vi "ReadTerminal.vi"(1 "reference":refnum<vi>) -> (0 "Terminal":T4)   [LabVIEW 2013]
uses:
  <vilib>/Utility/miscctls.llb/LVBoundsTypeDef.ctl
  <vilib>/Utility/miscctls.llb/LVRectTypeDef.ctl
  <vilib>/Utility/miscctls.llb/LVPositionTypeDef.ctl
panel:
  out "error out":errorcluster
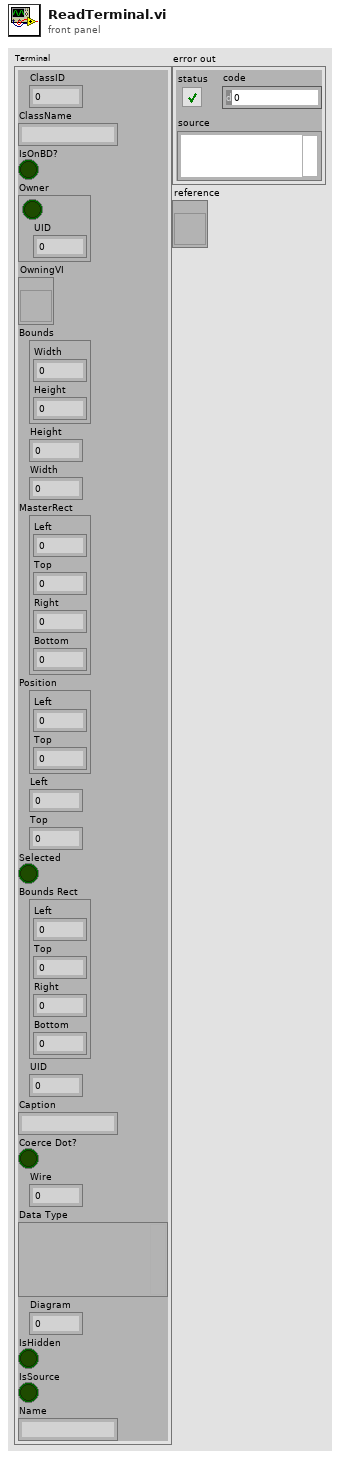
[diagram p1: front panel]
types:
  T1 = typedef "LVBoundsTypeDef.ctl" = cluster{"Width":u32, "Height":u32}
  T2 = typedef "LVRectTypeDef.ctl" = cluster{"Left":i16, "Top":i16, "Right":i16, "Bottom":i16}
  T3 = typedef "LVPositionTypeDef.ctl" = cluster{"Left":i32, "Top":i32}
  T4 = cluster{"ClassID":u32, "ClassName":string, "IsOnBD?":bool, "Owner":cluster{bool, "UID":i32}, "OwningVI":refnum<vi>, "Bounds":T1, "Height":u32, "Width":u32, "MasterRect":T2, "Position":T3, "Left":i32, "Top":i32, "Selected":bool, "Bounds Rect":T2, "UID":i32, "Caption":string, "Coerce Dot?":bool, "Wire":i32, "Data Type":variant, "Diagram":i32, "IsHidden":bool, "IsSource":bool, "Name":string}
  T5 = cluster{"ClassID":u32, "ClassName":string, "IsOnBD?":bool, "Cluster":cluster{bool, "UID":i32}, "OwningVI":refnum<vi>, "Bounds":T1, "Height":u32, "Width":u32, "MasterRect":T2, "Position":T3, "Left":i32, "Top":i32, "Selected":bool, "Bounds Rect":T2, "UID":i32, "Caption":string, "Coerce Dot?":bool, "UID":i32, "Data Type":variant, "UID":i32, "IsHidden":bool, "IsSource":bool, "Name":string}
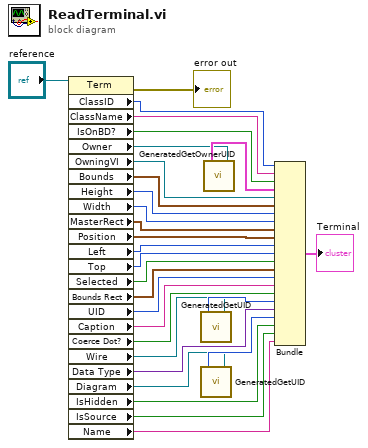
[diagram p0: block diagram]
diagram:
  n1 = property class="Term"(reference="reference") -> (error out=→"error out":errorcluster, "ClassID"=w28:u32, "ClassName"=w27:string, "IsOnBD?"=w26:bool, "Owner"=w24:refnum<vi>, "OwningVI"=w23:refnum<vi>, "Bounds"=w22:T1, "Height"=w21:u32, "Width"=w20:u32, "MasterRect"=w19:T2, "Position"=w18:T3, "Left"=w17:i32, "Top"=w16:i32, "Selected"=w15:bool, "Bounds Rect"=w14:T2, "UID"=w13:i32, "Caption"=w12:string, "Coerce Dot?"=w11:bool, "Wire"=w9:refnum<vi>, "Data Type"=w8:variant, "Diagram"=w6:refnum<vi>, "IsHidden"=w5:bool, "IsSource"=w4:bool, "Name"=w3:string)  [unwired: 1 in, 1 out]
  n2 = call "GeneratedGetUID.vi"("Text in"=w9) -> ("UID"=w10:i32)
  n3 = call "GeneratedGetUID.vi"("Text in"=w6) -> ("UID"=w7:i32)
  n4 = call "GeneratedGetOwnerUID.vi"("Generic in"=w24) -> ("Cluster"=w25:cluster{bool, "UID":i32})
  n5 = Bundle("ClassID"=w28, "ClassName"=w27, "IsOnBD?"=w26, "Cluster"=w25, "OwningVI"=w23, "Bounds"=w22, "Height"=w21, "Width"=w20, "MasterRect"=w19, "Position"=w18, "Left"=w17, "Top"=w16, "Selected"=w15, "Bounds Rect"=w14, "UID"=w13, "Caption"=w12, "Coerce Dot?"=w11, "UID"=w10, "Data Type"=w8, "UID"=w7, "IsHidden"=w5, "IsSource"=w4, "Name"=w3) -> (→"Terminal":T5)  [unwired: 1 in]
